vi "SParmGUI.vi"(5 "error in (no error)":errorcluster) -> (16 "output cluster":T1, 19 "error out":errorcluster)   [LabVIEW 2018]
panel:
  in  "W/Cal?":bool=TRUE
  in  "stop":bool
  in  "OK Button":bool
  in  "Power Level":dbl=-20.0 format="%_3g"
  in  "Sweep Type":string(combo)="LINear"
  in  "IF BW":dbl=10000.0 format="%_3g"
  in  "Format":string(combo)="MLOGarithmic"
  in  "Autoscale?":bool=TRUE
  in  "Average?":bool=TRUE
  in  "Avg. Factor":i32=20
  in  "S22":bool
  in  "S21":bool=TRUE
  in  "S12":bool
  in  "S11":bool
  in  "Stop Frequency":dbl=2000000000.0 format="%_3g"
  in  "Start Frequency":dbl=1000000000.0 format="%_3g"
  # "S-Parameter Measurement Parameters"
  # "Measurement"
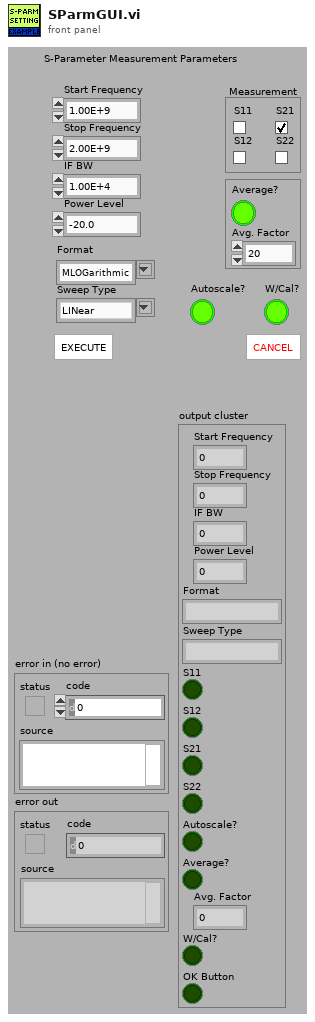
[diagram p1: front panel]
types:
  T1 = cluster{"Start Frequency":dbl, "Stop Frequency":dbl, "IF BW":dbl, "Power Level":dbl, "Format":string, "Sweep Type":string, "S11":bool, "S12":bool, "S21":bool, "S22":bool, "Autoscale?":bool, "Average?":bool, "Avg. Factor":i32, "W/Cal?":bool, "OK Button":bool}
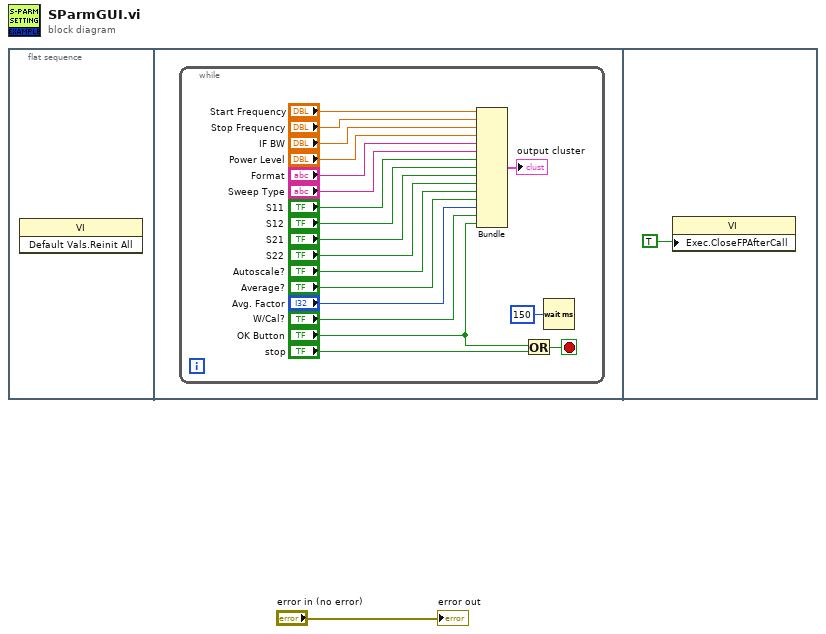
[diagram p0: block diagram]
diagram:
  n1 = flat-sequence {
    frame #0 {
      n2 = invoke class="VI" method="Default Vals.Reinit All"() -> ()  [unwired: 3 in, 3 out]
    }
    frame #1 {
      n3 = while {
        stop <- w6 stop-if-true
        n4 = Bundle("Start Frequency"="Start Frequency", "Stop Frequency"="Stop Frequency", "IF BW"="IF BW", "Power Level"="Power Level", "Format"="Format", "Sweep Type"="Sweep Type", "S11"="S11", "S12"="S12", "S21"="S21", "S22"="S22", "Autoscale?"="Autoscale?", "Average?"="Average?", "Avg. Factor"="Avg. Factor", "W/Cal?"="W/Cal?", "OK Button"="OK Button") -> (→"output cluster":T1)  [unwired: 1 in]
        n5 = Or(x="OK Button", y="stop") -> (x .or. y?=w6:bool)
        n6 = Wait (ms)(milliseconds to wait=u32 150) -> ()  [unwired: 1 out]
      }
    }
    frame #2 {
      n7 = property class="VI"("Exec.CloseFPAfterCall"=TRUE ("Execution:Close After Call")) -> ()  [unwired: 2 in, 2 out]
    }
  }
  "error out" <- "error in (no error)"
